vi "oa_Get DSA 9233 Oversample Rate and Filter Delay.vi"(11 "set sample rate":dbl) -> (0 "input delay":dbl, 1 "SampClkTimebase":dbl, 2 "Actual Sample Rate":dbl, 3 "oversample rate":dbl)   [LabVIEW 2017, in "SoundVib_TachProcess.lvlib"]
uses:
  <vilib>/addons/Sound and Vibration/Order Analysis/Tach Process/SoundVib_TachProcess.lvlib
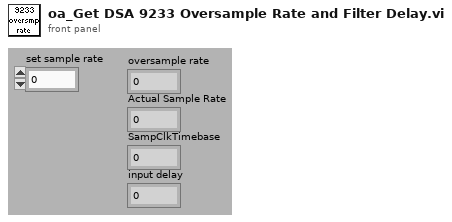
[diagram p1: front panel]
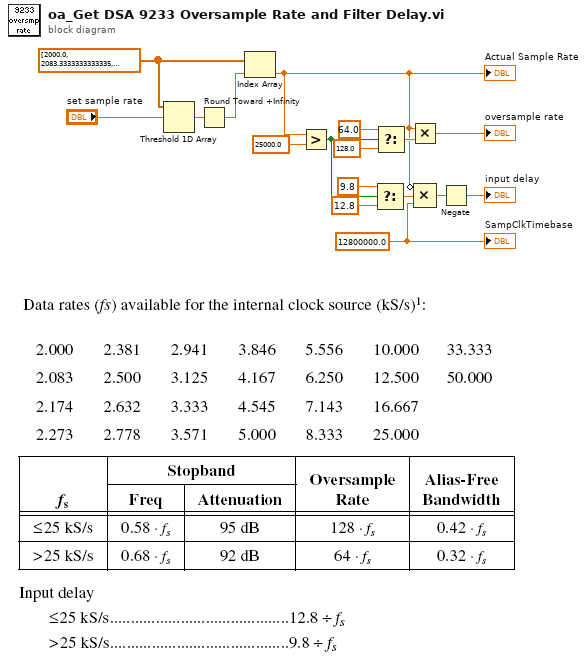
[diagram p0: block diagram]
diagram:
  w2 = 12800000.0 ("SampClkTimebase")
  w5 = dbl[] [2000.0, 2083.3333333333335, 2173.913043478261, 2272.7272727272725, 2380.9523809523807, 2500.0, 2631.5789473684213, 2777.777777777778, 2941.176470588235, 3125.0, 3333.3333333333335, 3571.4285714285716, 3846.153846153846, 4166.666666666667, 4545.454545454545, 5000.0, 5555.555555555556, 6250.0, 7142.857142857143, 8333.333333333334, 10000.0, 12500.0, 16666.666666666668, 25000.0, 33333.333333333336, 50000.0] ("reversed array")
  n1 = Threshold 1D Array(2:"set sample rate", 3:w5) -> (0:w17:dbl)  [unwired: 1 in]
  n2 = Round Toward +Infinity(x=w17) -> (ceil(x): smallest int >= x=w16:dbl)
  n3 = Index Array(array=w5, index=w16) -> (element=w1:dbl)
  "Actual Sample Rate" <- w1
  n4 = Greater?(x=w1, y=25000.0) -> (0:w10:bool)
  n5 = Select(t=9.8, s=w10, f=12.8) -> (s? t:f=w7:dbl)
  n6 = Select(t=64.0, s=w10, f=128.0) -> (s? t:f=w6:dbl)
  n7 = Multiply(x=w1, y=w6) -> (x*y=→"oversample rate":dbl)
  n8 = Compound Arithmetic op=MULTIPLY(invert w1, w7, w2) -> (w4:dbl)
  n9 = Negate(x=w4) -> (-x=→"input delay":dbl)
  "SampClkTimebase" <- w2
